vi "TIFF ULS Parameters.vi"(8 "error in (no error)":errorcluster, 10 "IFD":refnum<class "IFD.lvclass">, 11 "TIFF in":refnum<class "TIFF ULS.lvclass">) -> (0 "error out":errorcluster, 3 "TIFF out":refnum<class "TIFF ULS.lvclass">)   [LabVIEW 2016, in "TIFF ULS.lvclass"]
uses:
  TIFF ULS.lvclass
  IFD/IFD.lvclass
  TIFF ULS.lvclass/TIFF ULS.ctl
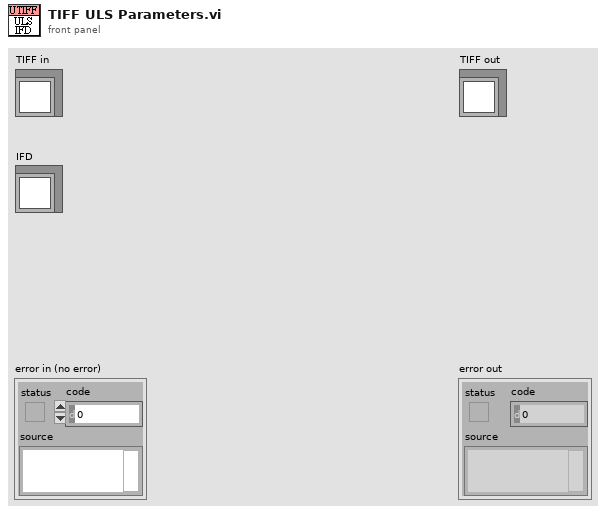
[diagram p1: front panel]
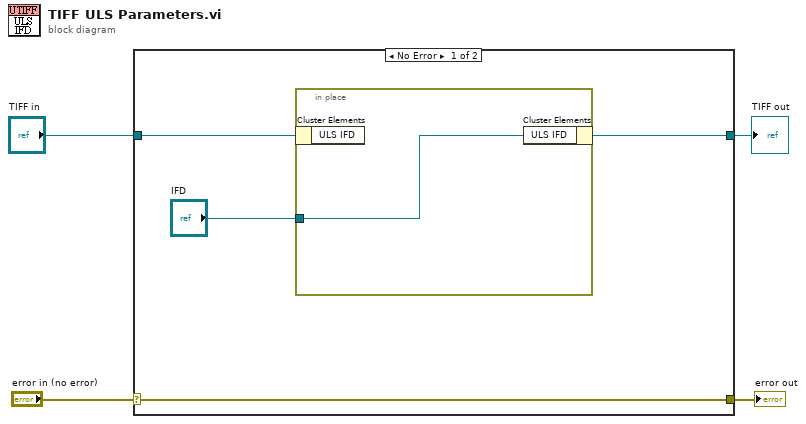
[diagram p0: block diagram]
diagram:
  n1 = case shown="No Error" "error in (no error)" {
    selector: "error in (no error)" -> [w8 w11]
    tunnel: [w8 w11] -> w3
    tunnel: [w5 w10] -> w1
    tunnel: "TIFF in" -> [w7 w10]
    frame No Error {
      n2 = in-place {
        in-place-border: "IFD" -> [w9]
        n3 = in-place-cluster #1(w7) -> ()  [unwired: 1 out]
        n4 = in-place-cluster #1("ULS IFD"=w9) -> (w5:refnum<class "TIFF ULS.lvclass">)
      }
    }
    frame Error {
    }
  }
  "error out" <- w3
  "TIFF out" <- w1
